vi "Configure DAQ.vi"(0 "System":T2={"System Type"=enum."DAQ Cart", "Serial Number"=0, "ID"="", "Cal File?"=FALSE}, 1 "Cal Files Path":path, 2 "Call By Refs":T1, 4 "Config":T5={"DAQ Settings"={"Trigger Type"=enum."Manual", "Trigger Samples"=0, "Pretrigger Samples"=0, "Trigger Interval"=0.0, "Time Units"=FALSE, "Auto Save"=FALSE, "Sample Rate"=7.0, "Select Analog"=FALSE, "Trigger Value"=0.0, "Trigger Stop Method"=enum."Use Samples Value to Stop Trigger", "Rate Sec/Min"=FALSE, "Save Mode"=enum."Single File", "File Size Limit"=0.0, "Log File Type"=enum."Basic", "Trigger Data Index"=0}, "Channels"=[], "Header"={"TA Number"="", "Test Name"="", "Serial Number"="", "Technician"=""}, "Graph Settings"={"Graph Labels"=[], [], [], [], [], [], [], [], [], [], [], [], [], "Graph Toggles"=[], "Axis Toggles"=[], "Graph Range"=enum."1"}, "Test Limits"=[], "All Type Info"=[], "Save Mode"=enum."Single File"} {"DAQ Settings"."Trigger Interval" min=0.0; "DAQ Settings"."Pretrigger Samples" min=0; "DAQ Settings"."Trigger Samples" min=0}, 5 "Channel Filter":bool[](array[boolean])=[FALSE, TRUE, TRUE, TRUE, TRUE, TRUE, TRUE, TRUE, TRUE, TRUE, TRUE, TRUE, TRUE, TRUE, TRUE, TRUE, TRUE, TRUE, TRUE, TRUE, TRUE, TRUE, TRUE, TRUE, TRUE, TRUE, TRUE, TRUE, TRUE, TRUE, TRUE, TRUE, TRUE, TRUE, TRUE, TRUE, TRUE, TRUE, TRUE, TRUE, TRUE, TRUE, TRUE, TRUE, TRUE, TRUE, TRUE, TRUE, TRUE], 7 "Sensor (scaling)":T4(array[cluster]), 8 "Manual/Timed Trigger":bool, 9 "Mode":enum16{"Init", "Acquire", "Clear"}(ring), 13 "CPU Saver Mode":bool, 14 "Total Channel Count":i16, 15 "Time Offset":dbl) -> (16 "Pretrigger Size":i32, 17 "scan rate":sgl=25.0, 18 "nx-5000 Mode:":string, 19 "Ntwk Sys Conn?":bool, 20 "Input Task OUT":refnum<k21>, 21 "Acquiring Data":bool, 22 "DO Task OUT":refnum<k21>, 23 "Freq Coefficients":cluster{"Coefficients":dbl[]}[](array[cluster]), 24 "DAQ Complete Trigger":bool, 25 "Data":sgl[][](array[numeric]), 26 "DI Task OUT":refnum<k21>, 27 "error out":errorcluster={"status"=TRUE, "code"=-10621, "source"="AI Control"})   [LabVIEW 2019]
uses:
  Type Defs and Controls/DAQ Settings.ctl
  Type Defs and Controls/Channel Config.ctl
  Type Defs and Controls/Header.ctl
  Type Defs and Controls/Sensor Config.ctl
  Type Defs and Controls/Trigger Stop Method.ctl
  Type Defs and Controls/Graph Settings Type Def.ctl
  Type Defs and Controls/Test Limits.ctl
  Type Defs and Controls/Part Info.ctl
  Type Defs and Controls/All Part Info.ctl
  Type Defs and Controls/Log File Type.ctl
  Type Defs and Controls/System Type.ctl
  Type Defs and Controls/Registered System.ctl
  Type Defs and Controls/Call By Refs.ctl
panel:
  out "Acquiring Data":bool
  # "EGU"
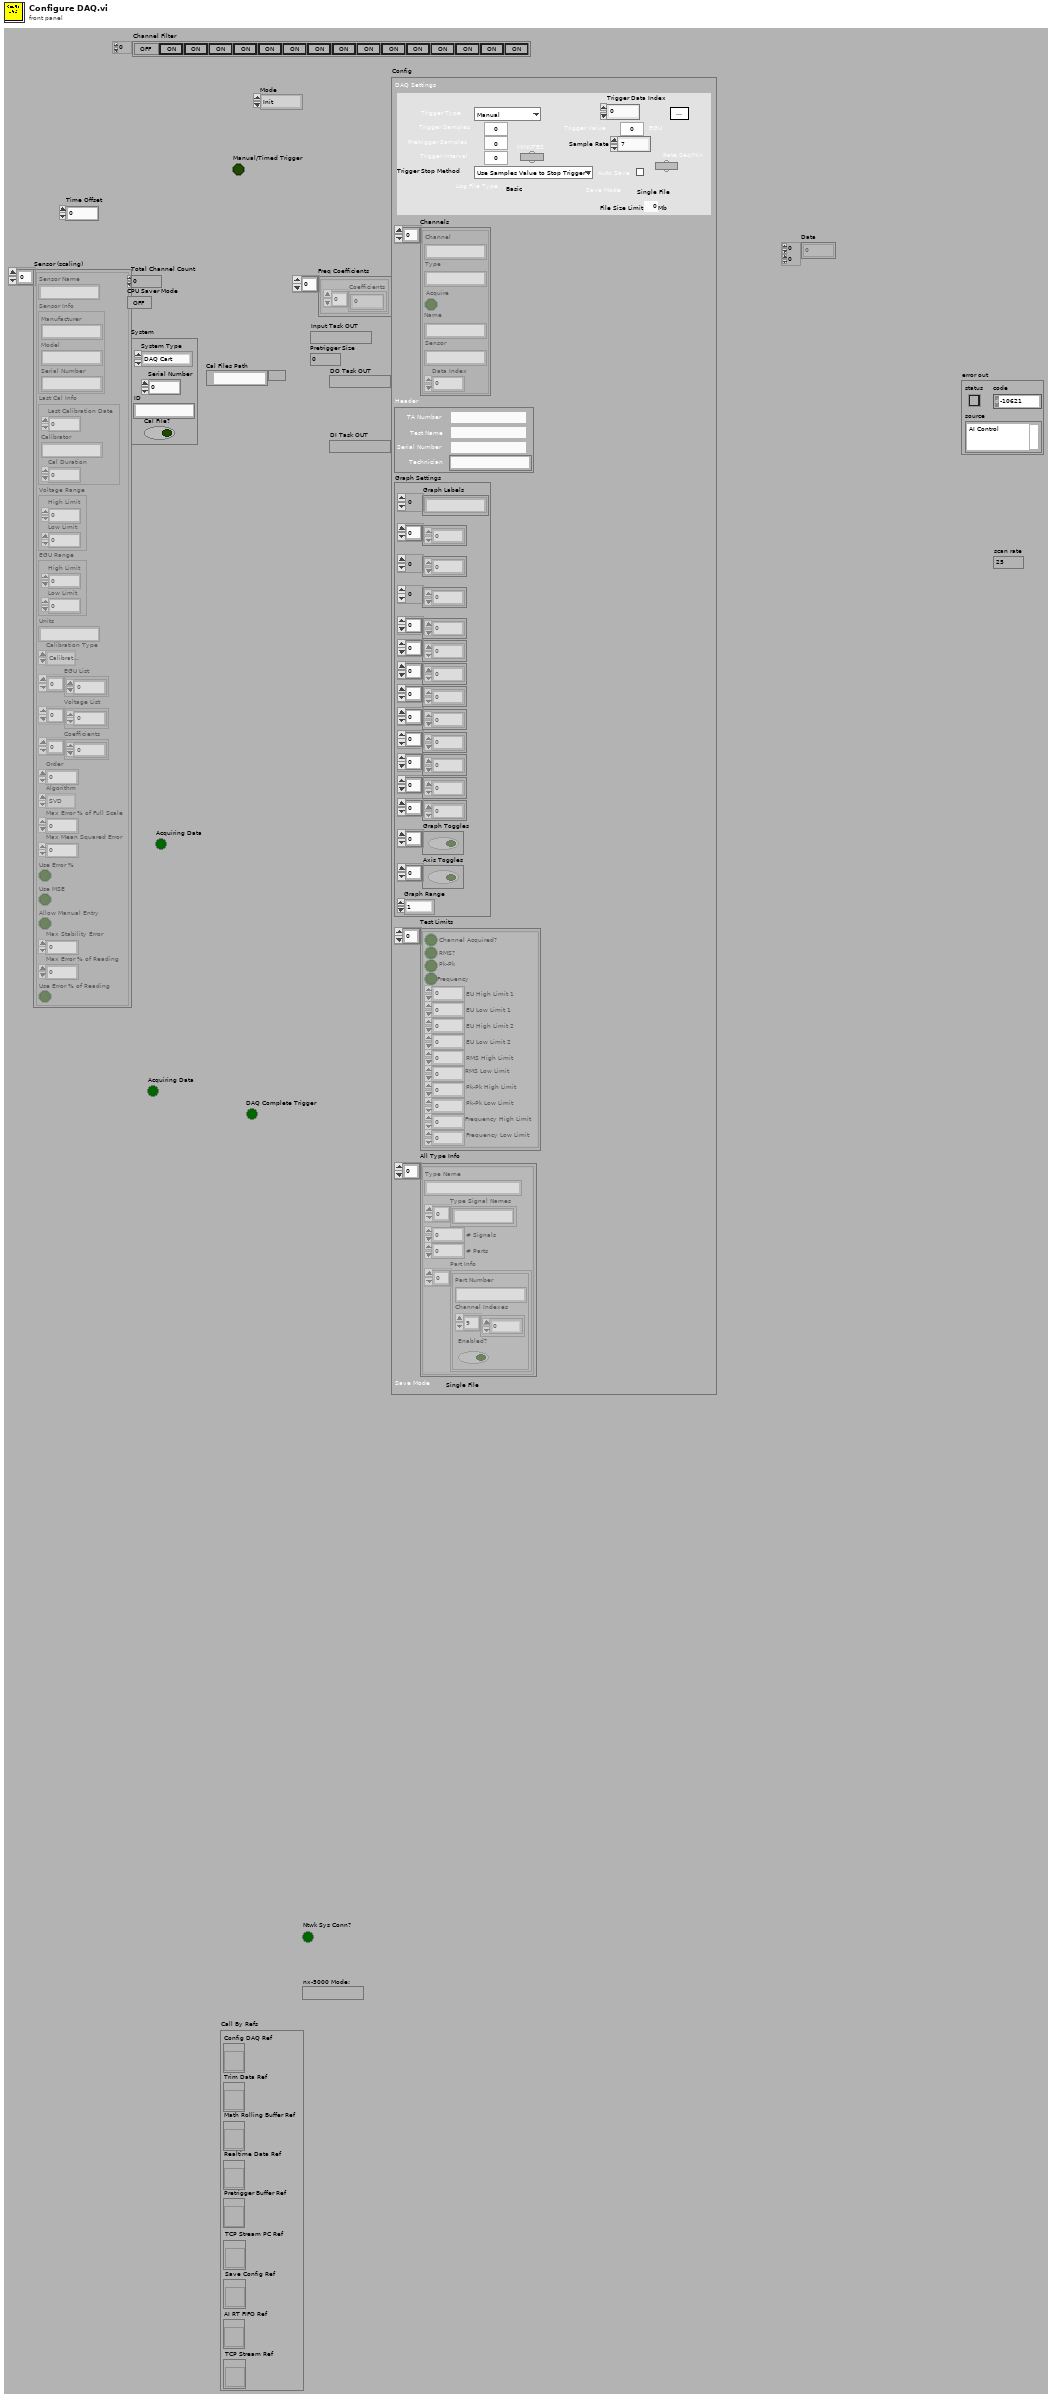
[diagram p1: front panel]
types:
  T1 = typedef "Call By Refs.ctl" = cluster{"Config DAQ Ref":refnum<vi>, "Trim Data Ref":refnum<vi>, "Math Rolling Buffer Ref":refnum<vi>, "Realtime Data Ref":refnum<vi>, "Pretrigger Buffer Ref":refnum<vi>, "TCP Stream PC Ref":refnum<vi>, "Save Config Ref":refnum<vi>, "AI RT FIFO Ref":refnum<vi>, "TCP Stream Ref":refnum<vi>}
  T2 = typedef "Registered System.ctl" = cluster{"System Type":T3, "Serial Number":u32, "ID":string, "Cal File?":bool}
  T3 = typedef "System Type.ctl" = enum16{"DAQ Rack", "DAQ Cart", "nx-5000", "unknown", "open"}
  T4 = cluster{"Sensor Name":string, "Sensor Info":cluster{"Manufacturer":string, "Model":string, "Serial Number":string}, "Last Cal Info":cluster{"Last Calibration Date":dbl, "Calibrator":string, "Cal Duration":i32}, "Voltage Range":cluster{"High Limit":dbl, "Low Limit":dbl}, "EGU Range":cluster{"High Limit":dbl, "Low Limit":dbl}, "Units":string, "Calibration Type":enum16{"Calibrate Analog", "Compare Analog Calibration"}, "EGU List":dbl[], "Voltage List":dbl[], "Coefficients":dbl[], "Order":i32, "Algorithm":enum32{"SVD", "Givens", "Givens2", "Householder", "LU Decomposition", "Cholesky"}, "Max Error % of Full Scale":dbl, "Max Mean Squared Error":dbl, "Use Error %":bool, "Use MSE":bool, "Allow Manual Entry":bool, "Max Stability Error":dbl, "Max Error % of Reading":dbl, "Use Error % of Reading":bool}[]
  T5 = typedef "Sensor Config.ctl" = cluster{"DAQ Settings":T6, "Channels":T9[], "Header":T10, "Graph Settings":T11, "Test Limits":T12[], "All Type Info":T13, "Save Mode":enum16{"Single File", "Segmented Files", "New File at Midnight"}}
  T6 = typedef "DAQ Settings.ctl" = cluster{"Trigger Type":enum16{"Manual", "Timed", "Analog Rising", "Analog Falling"}, "Trigger Samples":i32, "Pretrigger Samples":i32, "Trigger Interval":dbl, "Time Units":bool, "Auto Save":bool, "Sample Rate":dbl, "Select Analog":bool, "Trigger Value":dbl, "Trigger Stop Method":T7, "Rate Sec/Min":bool, "Save Mode":enum16{"Single File", "Segmented Files", "New File at Midnight"}, "File Size Limit":dbl, "Log File Type":T8, "Trigger Data Index":u32}
  T7 = typedef "Trigger Stop Method.ctl" = enum16{"Use Samples Value to Stop Trigger", "Use Threshold to Stop Trigger"}
  T8 = typedef "Log File Type.ctl" = enum16{"Basic", "RTS"}
  T9 = typedef "Channel Config.ctl" = cluster{"Channel":string, "Type":string, "Acquire":bool, "Name":string, "Sensor":string, "Data Index":u32}
  T10 = typedef "Header.ctl" = cluster{"TA Number":string, "Test Name":string, "Serial Number":string, "Technician":string}
  T11 = typedef "Graph Settings Type Def.ctl" = cluster{"Graph Labels":string[], u8[], i16[], u32[], u8[], u8[], u8[], u32[], u8[], u8[], u8[], dbl[], dbl[], "Graph Toggles":bool[], "Axis Toggles":bool[], "Graph Range":enum16{"1", "2", "3", "4", "5", "10", "15", "30", "60"}}
  T12 = typedef "Test Limits.ctl" = cluster{"Channel Acquired?":bool, "RMS?":bool, "Pk-Pk":bool, "Frequency":bool, "EU High Limit 1":dbl, "EU Low Limit 1":dbl, "EU High Limit 2":dbl, "EU Low Limit 2":dbl, "RMS High Limit":dbl, "RMS Low Limit":dbl, "Pk-Pk High Limit ":dbl, "Pk-Pk Low Limit":dbl, "Frequency High Limit":dbl, "Frequency Low Limit":dbl}
  T13 = typedef "All Part Info.ctl" = cluster{"Type Name":string, "Type Signal Names":string[], "# Signals":i32, "# Parts":i32, "Part Info":T14[]}[]
  T14 = typedef "Part Info.ctl" = cluster{"Part Number":string, "Channel Indexes":u16[], "Enabled?":bool}
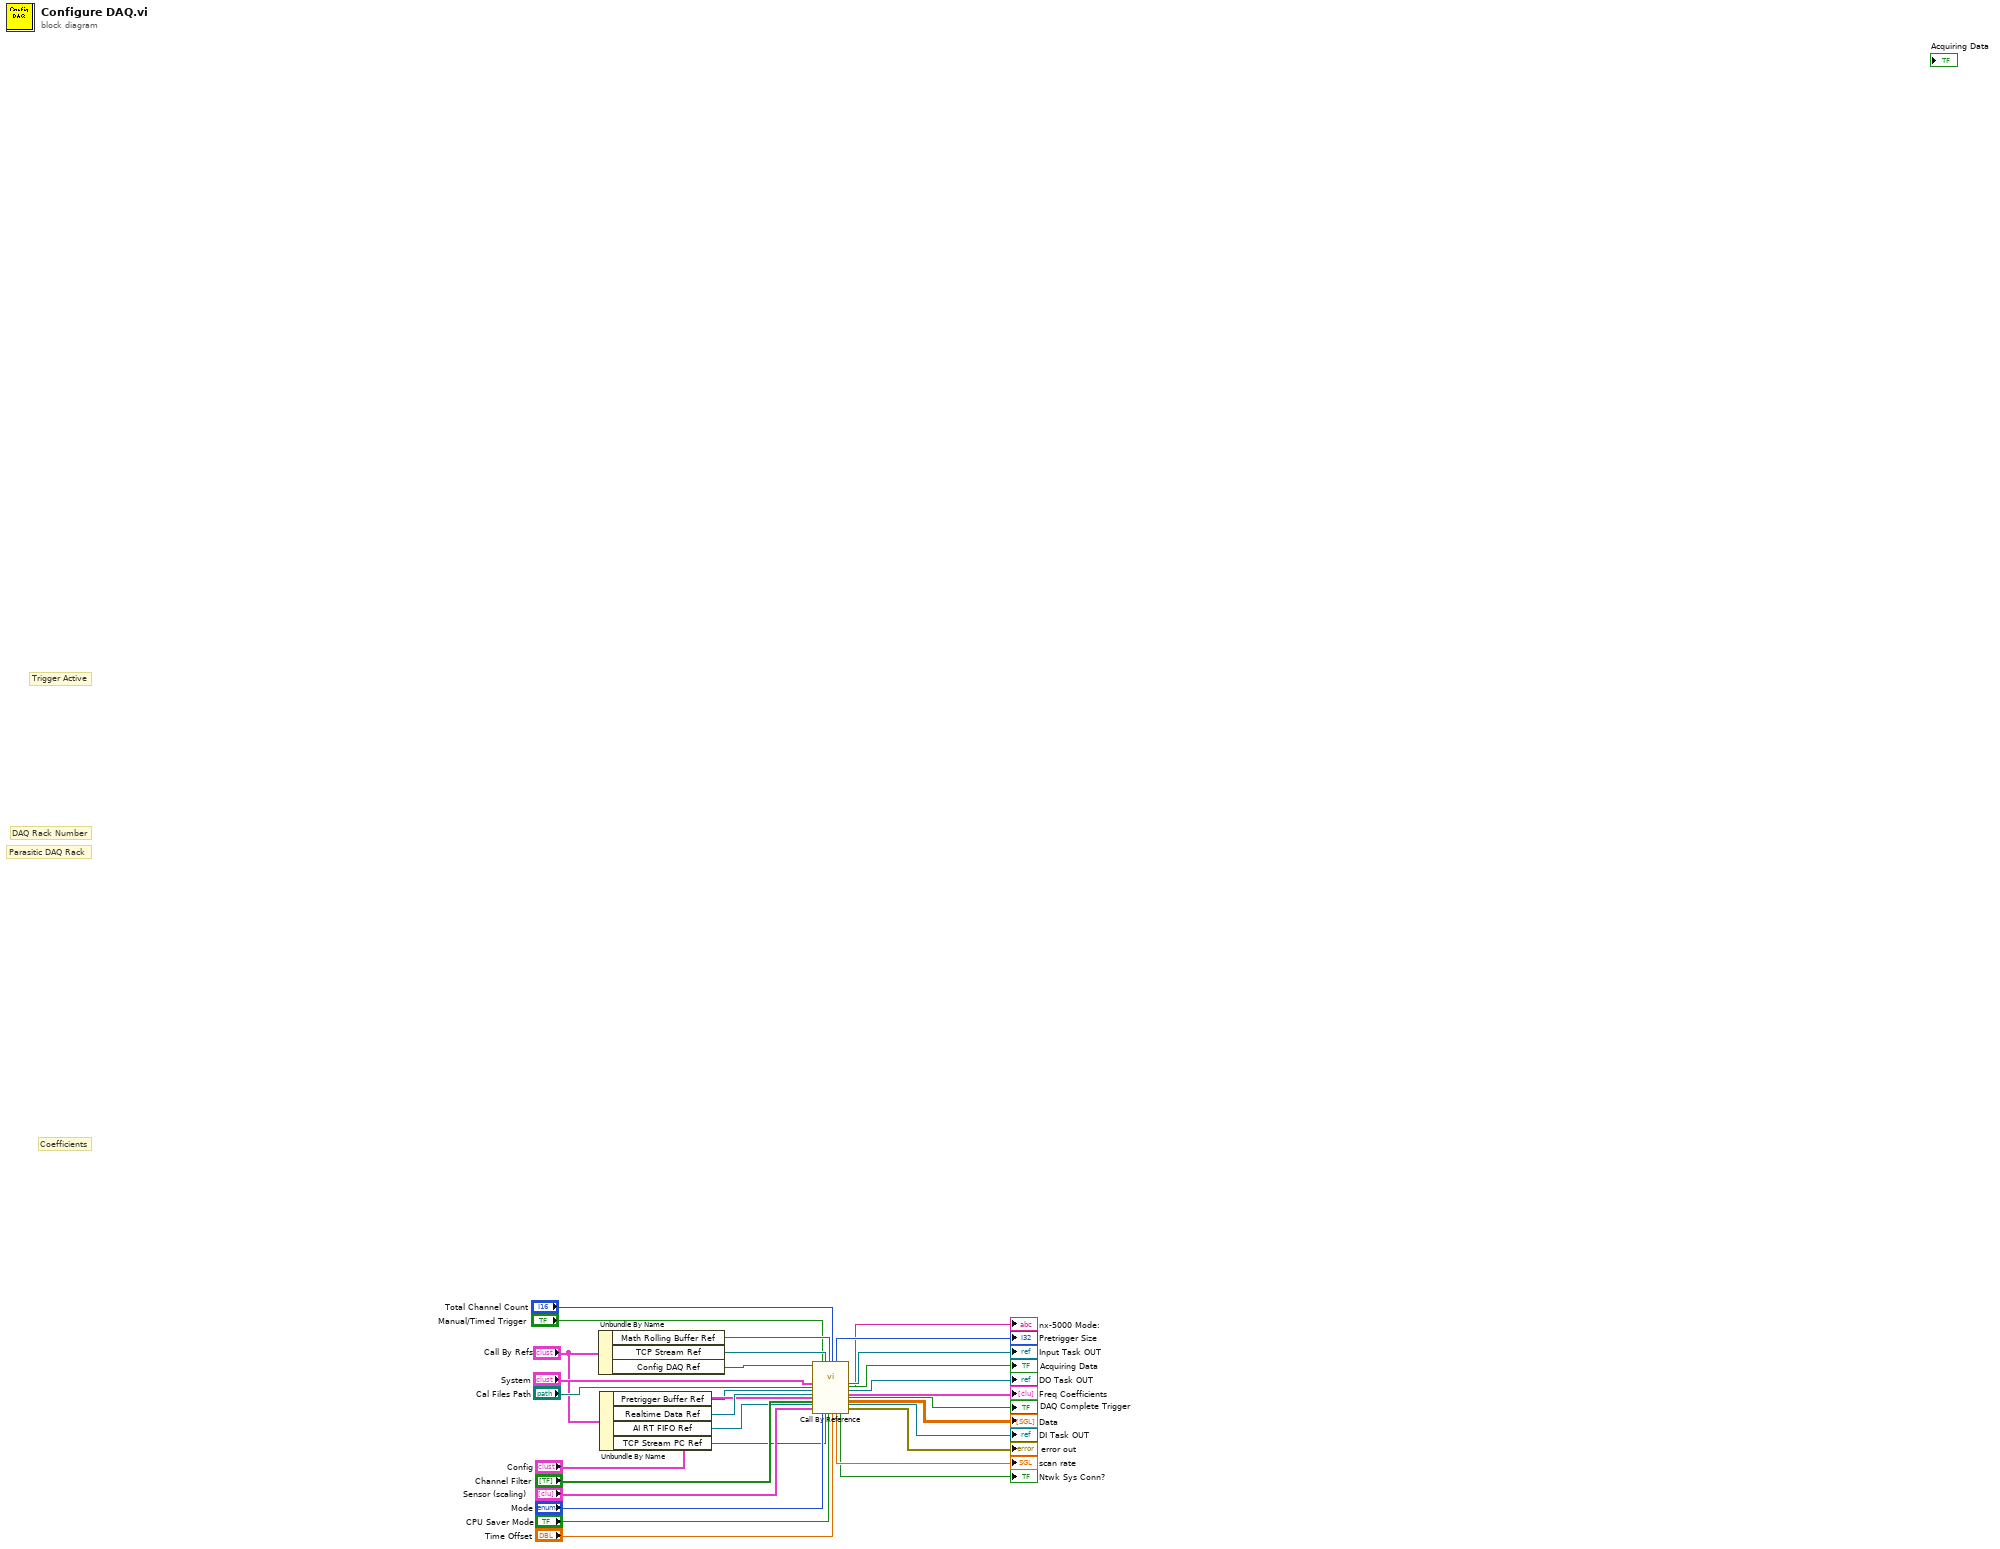
[diagram p0: block diagram]
diagram:
  # "Parasitic DAQ Rack"
  # "DAQ Rack Number"
  # "Coefficients"
  # "Trigger Active"
  n1 = Unbundle By Name("Call By Refs") -> ("Math Rolling Buffer Ref"=w26:refnum<vi>, "TCP Stream Ref"=w27:refnum<vi>, "Config DAQ Ref"=w28:refnum<vi>)
  n2 = Unbundle By Name("Call By Refs") -> ("Pretrigger Buffer Ref"=w2:refnum<vi>, "Realtime Data Ref"=w24:refnum<vi>, "AI RT FIFO Ref"=w5:refnum<vi>, "TCP Stream PC Ref"=w1:refnum<vi>)
  n3 = call-by-ref "?"(reference=w28, "System"="System", "Cal Files Path"="Cal Files Path", "Pretrigger Buffer Ref"=w2, "Realtime Data Ref"=w24, "Config"="Config", "Channel Filter"="Channel Filter", "AI RT FIFO Ref"=w5, "Sensor (scaling)"="Sensor (scaling)", "Manual/Timed Trigger"="Manual/Timed Trigger", "Mode"="Mode", "TCP Stream Ref"=w27, "TCP Stream PC Ref"=w1, "Math Rolling Buffer Ref"=w26, "CPU Saver Mode"="CPU Saver Mode", "Total Channel Count"="Total Channel Count", "Time Offset"="Time Offset") -> ("Pretrigger Size"=→"Pretrigger Size":i32, "scan rate"=→"scan rate":sgl, "nx-5000 Mode:"=→"nx-5000 Mode:":string, "Ntwk Sys Conn?"=→"Ntwk Sys Conn?":bool, "Input Task OUT"=→"Input Task OUT":refnum<k21>, "Acquiring Data"=→"Acquiring Data":bool, "DO Task OUT"=→"DO Task OUT":refnum<k21>, "Freq Coefficients"=→"Freq Coefficients":cluster{"Coefficients":dbl[]}[], "DAQ Complete Trigger"=→"DAQ Complete Trigger":bool, "Data"=→"Data":sgl[][], "DI Task OUT"=→"DI Task OUT":refnum<k21>, "error out"=→"error out":errorcluster)  [unwired: 1 in, 2 out]
